vi "Main.vi"(8 "error in (no error)":errorcluster, 9 "application reference":refnum<vi>, 10 "LabVIEW Object":refnum<class>) -> (0 "error out":errorcluster)   [LabVIEW 2018, in "DVR Accessor Library.lvlib"]
uses:
  DVR Accessor Library.lvlib
panel:
  # "Run Me!!!"
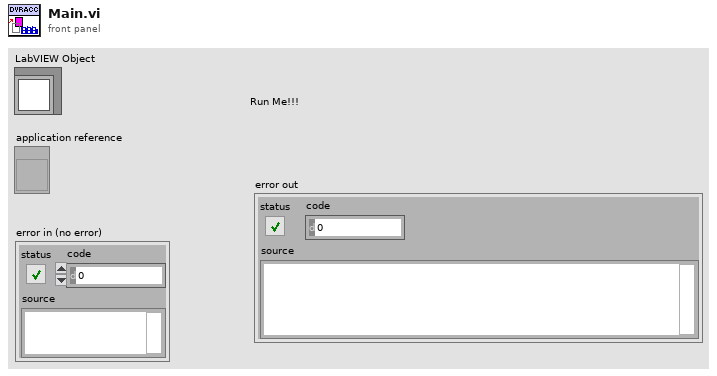
[diagram p1: front panel]
types:
  T1 = enum32{"invalid execution system", "user interface", "standard", "instrument i/o", "data acquisition", "other 1", "other 2", "same as caller"}
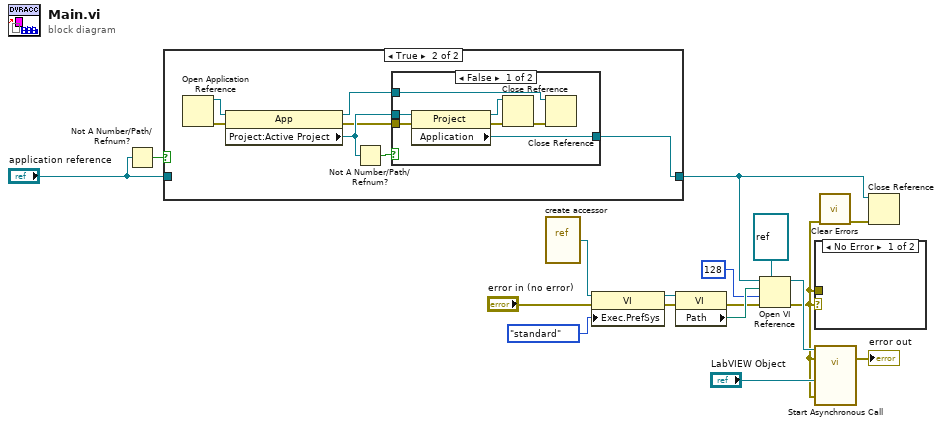
[diagram p0: block diagram]
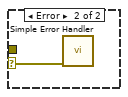
[diagram p4: hidden frame]
diagram:
  n1 = Not A Number/Path/Refnum?(number/path/refnum="application reference") -> (NaN/Path/Refnum?=w2:bool)
  n2 = case shown="True" w2 {
    tunnel: [w18 w19] -> w5
    tunnel: "application reference" -> [w18 _]
    frame False {
    }
    frame True {
      n3 = Open Application Reference() -> (0:w24:errorcluster, 3:w25:refnum<vi>)  [unwired: 4 in]
      n4 = property class="App"(reference=w25, error in=w24) -> (reference out=w20:refnum<vi>, error out=w21:errorcluster, "Project:Active Project"=w22:refnum<vi>)
      n5 = Not A Number/Path/Refnum?(number/path/refnum=w22) -> (NaN/Path/Refnum?=w23:bool)
      n6 = case shown="False" w23 {
        tunnel: w21 -> [w32 _]
        tunnel: [w31 w33] -> w19
        tunnel: w22 -> [w30 _]
        tunnel: w20 -> [w29 w33]
        frame False {
          n7 = property class="Project"(reference=w30, error in=w32) -> (reference out=w26:refnum<vi>, error out=w28:errorcluster, "Application"=w31:refnum<vi>)
          n8 = Close Reference(reference=w26, error in (no error)=w28) -> (error out=w27:errorcluster)
          n9 = Close Reference(reference=w29, error in (no error)=w27) -> ()  [unwired: 1 out]
        }
        frame True {
        }
      }
    }
  }
  n10 = vi-ref "create accessor.vi"() -> (w13:refnum<vi>)
  n11 = property class="VI"(reference=w13, error in="error in (no error)", "Exec.PrefSys"=T1."standard" ("Execution:Preferred Exec System")) -> (reference out=w12:refnum<vi>, error out=w11:errorcluster)
  n12 = property class="VI"(reference=w12, error in=w11) -> (error out=w10:errorcluster, "Path"=w17:path)  [unwired: 1 out]
  n13 = Open VI Reference(type specifier VI Refnum (for type only)=refnum<vi> refnum, application reference (local)=w5, vi path=w17, options=128, error in (no error)=w10) -> (vi reference=w15:refnum<vi>, error out=w4:errorcluster)  [unwired: 1 in]
  n14 = case shown="No Error" w4 {
    selector: w4 -> [_ w34]
    tunnel: w4 -> [_ _]
    frame No Error {
    }
    frame Error {
      n15 = call <vilib>:"Simple Error Handler.vi"("error in (no error)"=w34) -> ()  [unwired: 4 in, 5 out]
    }
  }
  n16 = call-by-ref "Start Asynchronous Call"(reference=w15, error in=w4, 8:"error in (no error)"=w4, "LabVIEW Object"="LabVIEW Object") -> (error out=→"error out":errorcluster)  [unwired: 9 in, 2 out]
  n17 = call <vilib>:"Clear Errors.vi"("error in (no error)"=w4) -> ("error out"=w3:errorcluster)  [unwired: 5 in, 1 out]
  n18 = Close Reference(reference=w5, error in (no error)=w3) -> ()  [unwired: 1 out]
